vi "execute.vi"(8 "error in (no error)":errorcluster, 10 "Context in":refnum<class "Context.lvclass">, 11 "EnableCommand in":refnum<class "EnableCommand.lvclass">) -> (0 "error out":errorcluster, 2 "Context out":refnum<class "Context.lvclass">, 3 "EnableCommand out":refnum<class "EnableCommand.lvclass">)   [LabVIEW 2016, in "EnableCommand.lvclass"]
uses:
  EnableCommand.lvclass
  Context/Context.lvclass
  EnableCommand.lvclass/EnableCommand.ctl
  Context/Context.lvclass/Context.ctl
  Context/getModel.vi
  Context/setModel.vi
  Model/getState.vi
  States/State/State.lvclass
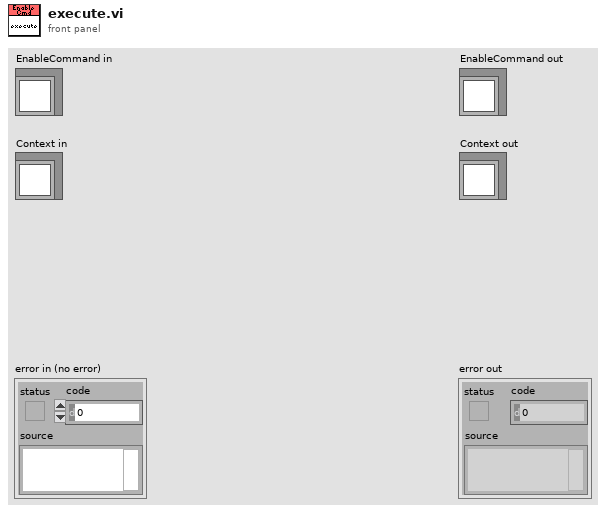
[diagram p1: front panel]
types:
  T1 = typedef "M1M3SupportTopics.lvlib/CommandEnable.ctl" = cluster{"CommandId":T2, "Enable":bool}
  T2 = typedef "M1M3SupportTopics.lvlib/CommandId.ctl" = i32
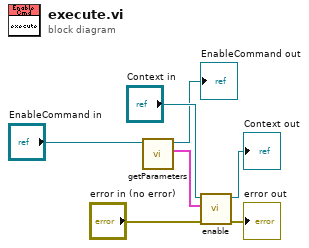
[diagram p0: block diagram]
diagram:
  n1 = call "getParameters.vi"("EnableCommand in"="EnableCommand in") -> ("Parameters"=w3:T1, "EnableCommand out"=→"EnableCommand out":refnum<class "EnableCommand.lvclass">)  [unwired: 9 in]
  n2 = call "enable.vi"("error in (no error)"="error in (no error)", "Parameters"=w3, "Context in"="Context in") -> ("error out"=→"error out":errorcluster, "Context out"=→"Context out":refnum<class "Context.lvclass">)  [unwired: 7 in]
